vi "GetFunctionArbs.vi"(8 "error in (no error)":errorcluster, 11 "PmuTestFunctions in":refnum<class "PmuTestFunctions.lvclass">) -> (0 "error out":errorcluster, 2 "Arbs":variant, 3 "PmuTestFunctions out":refnum<class "PmuTestFunctions.lvclass">)   [LabVIEW 2018, in "Functions.lvlib" / "PmuTestFunctions.lvclass"]
uses:
  PmuTestFunctions.lvclass
  X:/Projects/PMUCal/Modules/FGen/MemberClasses/ArbitraryFunction/ArbitraryFunction.lvclass
  ArbitraryFunction/ArbitraryFunction.lvclass/ArbitraryFunction.ctl
  PmuTestFunctions.lvclass/PmuTestFunctions.ctl
  ArbitraryFunction/TypeDefs/Arbs.ctl
  ArbitraryFunction/Accessors/Read SampleRate.vi
  Accessors/Read SettlingTime.vi
  Accessors/Read T0.vi
  ArbitraryFunction/Accessors/Read Arbs.vi
  ArbitraryFunction/ArbitraryFunction.lvclass
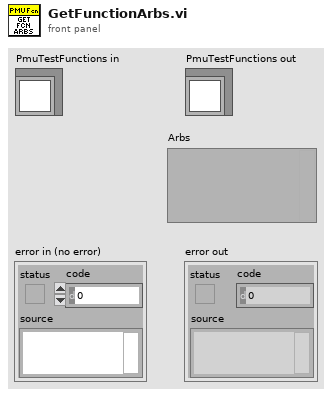
[diagram p1: front panel]
types:
  T1 = cluster{"Arbs":cluster{"Handle":string, "Size":i32, "Gain":dbl, "Offset":dbl}[], "SampleRate":dbl, "SettlingTime":dbl, "T0":dbl}
  T2 = typedef "Functions.lvlib/ArbitraryFunction.lvclass/Arbitrary.ctl" = cluster{"Handle":string, "Size":i32, "Gain":dbl, "Offset":dbl, "Waveform":waveform(dbl)}
  T3 = typedef "Functions.lvlib/ArbitraryFunction.lvclass/Arbs.ctl" = cluster{"Handle":string, "Size":i32, "Gain":dbl, "Offset":dbl}
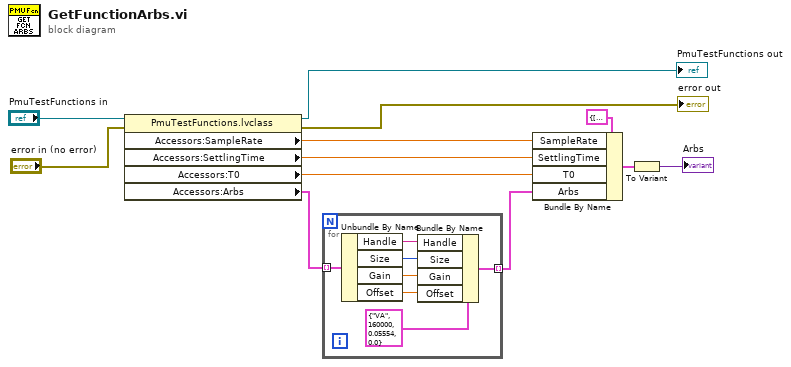
[diagram p0: block diagram]
diagram:
  n1 = property class="PmuTestFunctions.lvclass"(reference="PmuTestFunctions in", error in="error in (no error)") -> (reference out=→"PmuTestFunctions out":refnum<class "PmuTestFunctions.lvclass">, error out=→"error out":errorcluster, "Accessors:SampleRate"=w8:dbl, "Accessors:SettlingTime"=w7:dbl, "Accessors:T0"=w6:dbl, "Accessors:Arbs"=w10:T2[])
  n2 = for {
    tunnel: w10 -> [w19] mode=indexing
    tunnel: [w13] -> w5 mode=indexing
    n3 = Unbundle By Name(w19) -> ("Handle"=w17:string, "Size"=w16:i32, "Gain"=w15:dbl, "Offset"=w14:dbl)
    n4 = Bundle By Name(cluster=T3 {"Handle"="VA", "Size"=160000, "Gain"=0.05554, "Offset"=0.0} ("Arbs"), "Handle"=w17, "Size"=w16, "Gain"=w15, "Offset"=w14) -> (w13:T3)
  }
  n5 = Bundle By Name(cluster=T1 {"Arbs"=[], "SampleRate"=0.0, "SettlingTime"=0.0, "T0"=0.0} ("FunctionConfig"), "SampleRate"=w8, "SettlingTime"=w7, "T0"=w6, "Arbs"=w5) -> (w4:T1)
  n6 = To Variant(anything=w4) -> (Variant=→"Arbs":variant)
